vi "Configure Operation.vi"(8 "error in (no error)":errorcluster, 10 "Operation Mode (0:AC)":u32(ring) items=["AC", "DC", "AC+DC"], 11 "VISA resource name":refnum<visa-resource-name>) -> (0 "error out":errorcluster, 3 "VISA resource name out":refnum<visa-resource-name>)   [LabVIEW 2010, in "California Instruments iX Series.lvlib"]
doc: "Configures the operation mode of the instrument. The i series provides either AC or DC mode while the iX series adds AC+DC mode."
uses:
  <instrlib>/California Instruments iX Series/California Instruments iX Series.lvlib
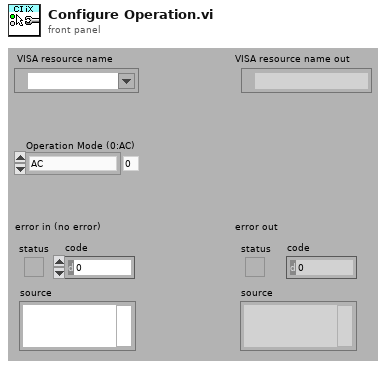
[diagram p1: front panel]
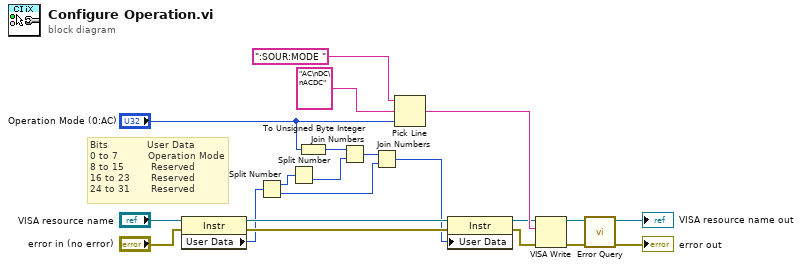
[diagram p0: block diagram]
diagram:
  # "Bits             User Data       \n0 to 7          Operation Mode\n8 to 15         Reserved\n16 to 23       Reserved\n24 to 31       Reserved"
  n1 = property class="Instr"(reference="VISA resource name", error in="error in (no error)") -> (reference out=w11:refnum<visa-resource-name>, error out=w10:errorcluster, "User Data"=w7:u32)
  n2 = Split Number(x=w7) -> (hi(x)=w5:u16, lo(x)=w2:u16)
  n3 = Split Number(x=w5) -> (lo(x)=w4:u8)  [unwired: 1 out]
  n4 = To Unsigned Byte Integer(number="Operation Mode (0:AC)") -> (unsigned 8bit integer=w6:u8)
  n5 = Join Numbers(hi=w6, lo=w4) -> ((hi.lo)=w3:u16)
  n6 = Join Numbers(hi=w3, lo=w2) -> ((hi.lo)=w1:u32)
  n7 = Pick Line(string ("")=":SOUR:MODE ", multi-line string="AC\nDC\nACDC", line index="Operation Mode (0:AC)") -> (output string=w15:string)
  n8 = property class="Instr"(reference=w11, error in=w10, "User Data"=w1) -> (reference out=w14:refnum<visa-resource-name>, error out=w13:errorcluster)
  n9 = VISA Write(VISA resource name=w14, write buffer=w15, error in (no error)=w13) -> (VISA resource name out=w19:refnum<visa-resource-name>, error out=w18:errorcluster)  [unwired: 1 out]
  n10 = call <instrlib>:"Error Query.vi"("error in (no error)"=w18, "VISA resource name"=w19) -> ("error out"=→"error out":errorcluster, "VISA resource name out"=→"VISA resource name out":refnum<visa-resource-name>)  [unwired: 6 in, 2 out]
